vi "Ballard - 1553 - Load Database.vi"(8 "error in (no error)":errorcluster, 11 "Node Ptr":u64 format="%.0x") -> (0 "error out":errorcluster)   [LabVIEW 2017, in "Ballard 1553 System Explorer.lvlib"]
uses:
  Ballard 1553 System Explorer.lvlib
  SubVIs/Create Sysdef Tree from DB Channel Clusters.vi
  Shared/Controls and Global/Global.vi
  <vilib>/NI Veristand/Custom Device API/Get Item Property (Path).vi
  SubVIs/Parse DB.vi
  <vilib>/NI Veristand/Custom Device API/NI VeriStand - Enable System Explorer Update Buffer.vi
  <vilib>/NI Veristand/Custom Device API/NI VeriStand - Add Custom Device Section.vi
  SubVIs/Create Sysdef Tree from DB Channel Clusters_BC.vi
  SubVIs/Create Sysdef Tree from DB Channel Clusters_RTs.vi
  <vilib>/NI Veristand/Custom Device API/NI VeriStand - Commit System Explorer Update Buffer.vi
  <vilib>/NI Veristand/Custom Device API/Set Item Property (Boolean).vi
  <vilib>/NI Veristand/Custom Device API/Set Item Property (String).vi
  <vilib>/NI Veristand/Custom Device API/Set Item Property (Path).vi
  <vilib>/NI VeriStand/Custom Device API/Custom Device API.lvlib
  <vilib>/NI VeriStand/Custom Device Tools/Custom Device Utility Library/Custom Device Utility Library.lvlib
  Shared/Ballard 1553 Shared.lvlib
panel:
  in  "Tag":string
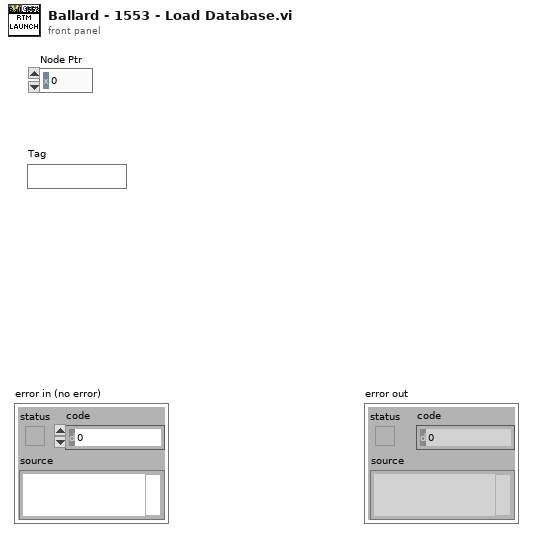
[diagram p1: front panel]
types:
  T1 = typedef "Custom Device API.lvlib/Custom Device Item Ref.ctl" = u64
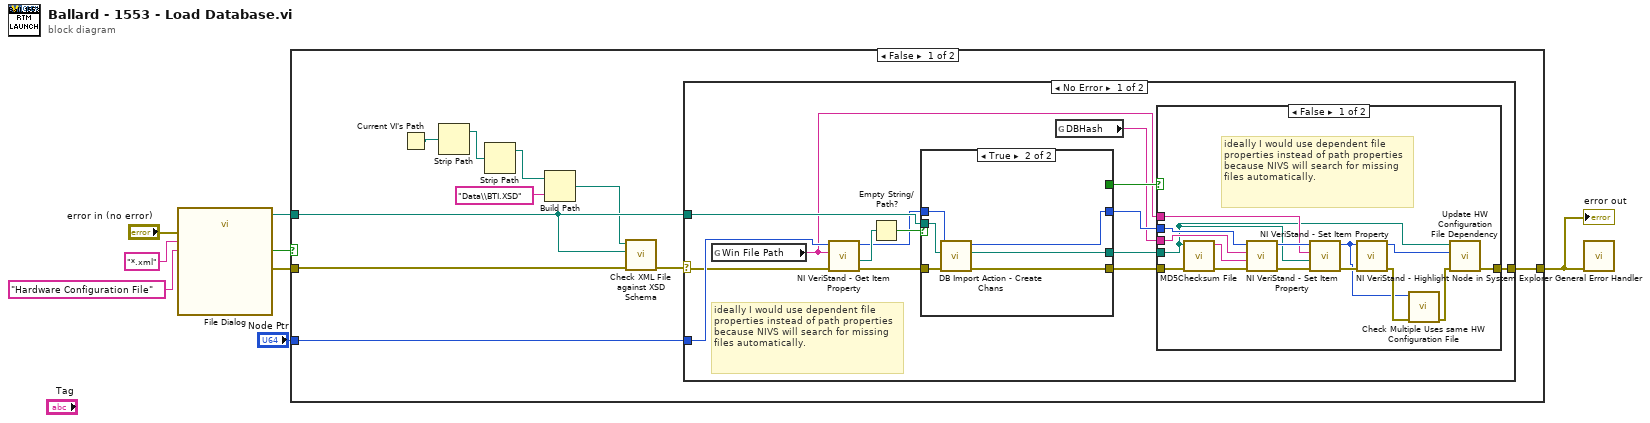
[diagram p0: block diagram]
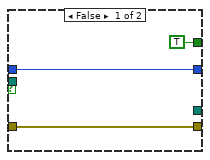
[diagram p3: hidden frame]
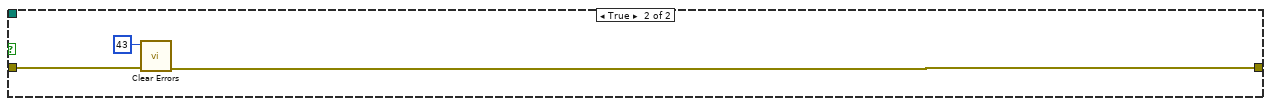
[diagram p5: hidden frame]
diagram:
  n1 = call "File Dialog"("error in"="error in (no error)", "pattern (all files)"="*.xml", "pattern label"="Hardware Configuration File") -> ("selected path"=w1:path, "cancelled"=w4:bool, "error out"=w3:errorcluster)  [unwired: 9 in, 1 out]
  n2 = case shown="False" w4 {
    tunnel: [w18 w59] -> w8
    tunnel: w3 -> [w15 w60]
    tunnel: "Node Ptr" -> [w17 _]
    tunnel: w1 -> [w14 _]
    frame False {
      n3 = Current VI's Path() -> (path=w11:path)
      n4 = Strip Path(path=w11) -> (stripped path=w12:path)  [unwired: 1 out]
      n5 = Strip Path(path=w12) -> (stripped path=w13:path)  [unwired: 1 out]
      n6 = Build Path(base path=w13, name or relative path="Data\\BTI.XSD") -> (appended path=w10:path)
      n7 = call "Check XML File against XSD Schema.vi"("error in (no error)"=w15, "XML Configuration File Path"=w14, "XML Schema File Path"=w10) -> ("error IO"=w16:errorcluster)  [unwired: 8 in]
      n8 = case shown="No Error" w16 {
        selector: w16 -> [w21 w58]
        tunnel: [w29 w58] -> w18
        tunnel: w17 -> [w28 _]
        tunnel: w14 -> [w25 _]
        frame No Error {
          # "ideally I would use dependent file properties instead of path properties because NIVS will search for missing files automatically."
          n9 = global read "Global.vi" "Win File Path"() -> (w20:string)
          n10 = call-poly <vilib>:"NI VeriStand - Get Item Property.vi"("error in (no error)"=w21, "Property Name"=w20, "Item Ref in"=w28) -> ("error out"=w22:errorcluster, "Value"=w26:path, "Item Ref out"=w23:T1)  [unwired: 5 in, 1 out]
          n11 = Empty String/Path?(string/path=w26) -> (empty?=w24:bool)
          n12 = case shown="True" w24 {
            tunnel: [w51 w57] -> w32
            tunnel: [w50 w56] -> w31
            tunnel: [_ w55] -> w30
            tunnel: w22 -> [w51 w54]
            tunnel: [TRUE ("Cancelled?") _] -> w27
            tunnel: w25 -> [_ w53]
            tunnel: w23 -> [w50 w52]
            frame False {
            }
            frame True {
              n13 = call "DB Import Action - Create Chans.vi"("error in (no error)"=w54, "selected path"=w53, "Node Ptr"=w52) -> ("error out"=w57:errorcluster, "selected path out"=w55:path, "Node Ptr dup"=w56:u64)  [unwired: 6 in]
            }
          }
          n14 = global read "Global.vi" "DBHash"() -> (w19:string)
          n15 = case shown="False" w27 {
            tunnel: w32 -> [w41 w48]
            tunnel: w31 -> [w47 _]
            tunnel: w30 -> [w37 _]
            tunnel: [w38 w48] -> w29
            tunnel: w19 -> [w43 _]
            tunnel: w20 -> [w42 _]
            frame False {
              # "ideally I would use dependent file properties instead of path properties because NIVS will search for missing files automatically."
              n16 = call <vilib>:"MD5Checksum File.vi"("error in (no error)"=w41, "Path"=w37) -> ("error out"=w40:errorcluster, "MD5 message-digest"=w39:string)  [unwired: 8 in]
              n17 = call-poly <vilib>:"NI VeriStand - Set Item Property.vi"("error in (no error)"=w40, "Value"=w39, "Property Name"=w43, "Item Ref in"=w47) -> ("error out"=w44:errorcluster, "Item Ref out"=w45:T1)  [unwired: 5 in, 1 out]
              n18 = call-poly <vilib>:"NI VeriStand - Set Item Property.vi"("error in (no error)"=w44, "Value"=w37, "Property Name"=w42, "Item Ref in"=w45) -> ("error out"=w46:errorcluster, "Item Ref out"=w33:T1)  [unwired: 5 in, 1 out]
              n19 = call <vilib>:"NI VeriStand - Highlight Node in System Explorer.vi"("error in (no error)"=w46, "Item Ref in"=w33) -> ("error out"=w35:errorcluster, "Node Ptr dup"=w36:T1)  [unwired: 8 in]
              n20 = call "Check Multiple Uses same HW Configuration File.vi"("error in (no error)"=w35, "Item Ref in"=w33) -> ("error out"=w34:errorcluster)  [unwired: 9 in]
              n21 = call "Update HW Configuration File Dependency.vi"("error in (no error)"=w34, "Node Ptr dup"=w36, "selected path in"=w37) -> ("error out"=w38:errorcluster)  [unwired: 8 in]
            }
            frame True {
            }
          }
        }
        frame Error {
        }
      }
    }
    frame True {
      n22 = call <vilib>:"Clear Errors.vi"("error in (no error)"=w60, "specific error code to clear (0: all)"=43) -> ("error out"=w59:errorcluster)  [unwired: 4 in, 1 out]
    }
  }
  "error out" <- w8
  n23 = call <vilib>:"General Error Handler.vi"("error in (no error)"=w8) -> ()  [unwired: 10 in, 5 out]
